vi "OpenLoftyDrve.vi"(8 "error in (no error)":errorcluster) -> (0 "error out":errorcluster)   [LabVIEW 2015]
uses:
  <vilib>/Rock Robotics/WPI/CAN/TalonSRX/WPI_CANTalonSRX_APIControlMode.ctl
  <vilib>/Rock Robotics/WPI/CAN/TalonSRX/WPI_CANTalonSRX_APIFeedbackSelect.ctl
  Advanced Drive VIs/PID Type Def.ctl
  RobotDriveGlobal.vi
  LED Lights/LED Lights Global.vi
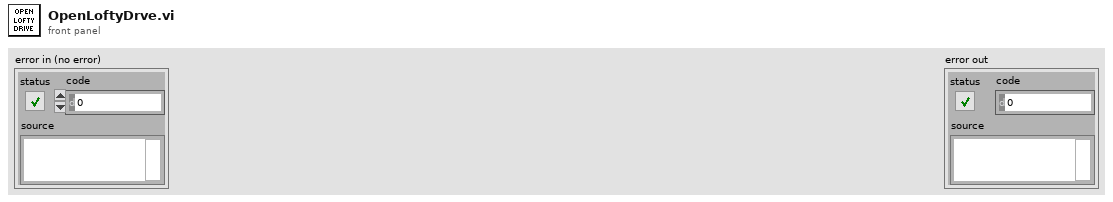
[diagram p1: front panel]
types:
  T1 = typedef "PID Type Def.ctl" = cluster{"P":dbl, "I":dbl, "D":dbl, "F":dbl, "I Zone":dbl, "Ramp Rate":dbl}
  T2 = typedef "WPI_CANTalonSRX_APIFeedbackSelect.ctl" = enum16{"Digital Quadrature Encoder", "Analog Potentiometer", "Analog Encoder", "Count on Quad-A (Rising-Edge)", "Count on Quad-A (Falling-Edge)", "CTR Magnetic Enc (Absolute)", "CTR Magnetic Enc (Relative)", "Pulse Width"}
  T3 = typedef "WPI_CANTalonSRX_APIControlMode.ctl" = enum8{"Percent VBus", "Speed", "Position", "Slave", "Unchanged / Invalid", "Voltage Compensation", "Current", "Motion Profile"}
  T4 = typedef "Drive Global Type Def.ctl" = cluster{"Left Drive Motors":T5, "Right Drive Motors":T5}
  T5 = typedef "Master Slave Drive Motors Type Def.ctl" = cluster{"Motor Front":T6, "Motor Back":T6, "Motor Errors":errorcluster, "Motor Top":T6, "Initialized":bool}
  T6 = typedef "Motor Global Type Def.ctl" = cluster{"Motor Error":errorcluster}
  T7 = typedef "WPI_MotorControlDeviceRef.ctl" = cluster{"DeviceStatus":errorcluster, "Type":T8, "PWM":cluster{"PWM Channel":T9, "DeadBand":T10}, "CAN":cluster{"Device Number":u8, "Control Mode":T11, "Semaphore":T12, "Max Vout":dbl, "TalonSRX Control Mode":T3}, "Invert":bool}
  T8 = typedef "WPI_MotorControlType.ctl" = enum16{"PWM", "CAN", "CANTalonSRX"}
  T9 = typedef "FPGA_DIOPWMChannel.ctl" = enum8{"PWM 0", "PWM 1", "PWM 2", "PWM 3", "PWM 4", "PWM 5", "PWM 6", "PWM 7", "PWM 8", "PWM 9", "PWM MXP 0", "PWM MXP 1", "PWM MXP 2", "PWM MXP 3", "PWM MXP 4", "PWM MXP 5", "PWM MXP 6", "PWM MXP 7", "PWM MXP 8", "PWM MXP 9", "Invalid"}
  T10 = typedef "WPI_PWMDeadband.ctl" = cluster{"Name":string, "maxPositivePwm":i32, "minPositivePwm":i32, "centerPwm":i32, "maxNegativePwm":i32, "minNegativePwm":i32, "angularRange":u16}
  T11 = typedef "WPI_CANJaguar_ControlMode.ctl" = enum8{"Percent VBus", "Current", "Speed", "Position", "Voltage"}
  T12 = typedef "Semaphore RefNum" = refnum<k1>
  T13 = typedef "RobotDrive Type Def.ctl" = cluster{"RobotDriveDevRef":cluster{"DevStatus":errorcluster, "Motors[]":T7[], "Square Inputs":bool, "Max Output":dbl}, "Control Mode":T3, "Motor Settings":T14, "Default Control Mode":T3, "Speed Mag":dbl}
  T14 = typedef "Drive Motor Settings.ctl" = cluster{"Wheel Radius":dbl, "Encoder Ticks Per Rev":dbl, "Gear Ratio":dbl, "ClimbRev":dbl}
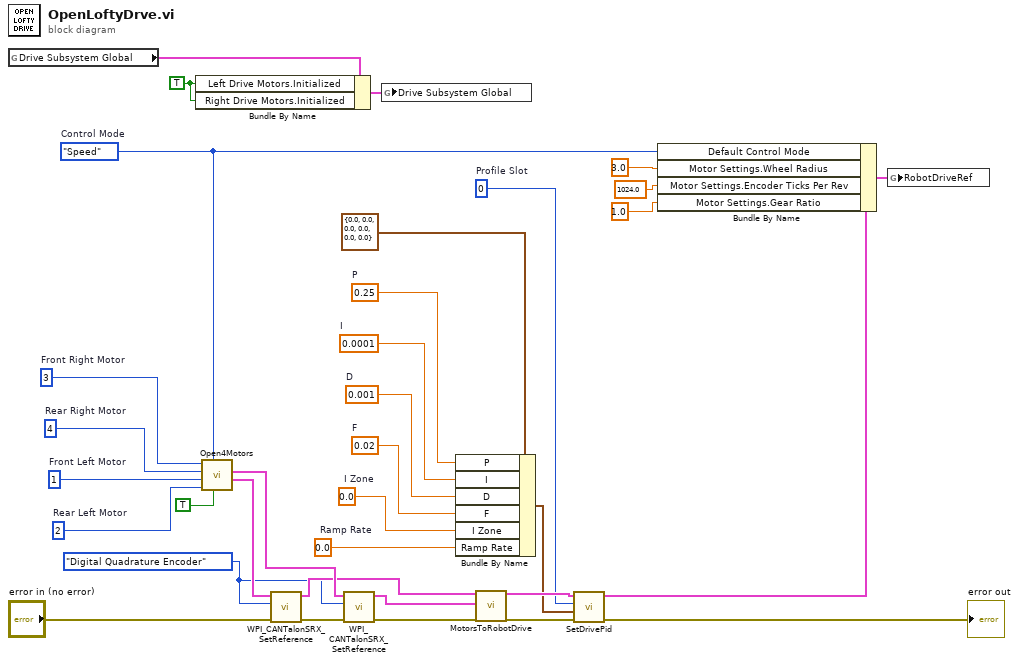
[diagram p0: block diagram]
diagram:
  w34 = TRUE
  w26 = u8 0  # Profile Slot
  w25 = 0.0  # Ramp Rate
  w24 = 0.0  # I Zone
  w23 = 0.02  # F
  w22 = 0.001  # D
  w21 = 0.0001  # I
  w20 = 0.25  # P
  w7 = WPI_CANTalonSRX_APIFeedbackSelect."Digital Quadrature Encoder" ("Feedback Reference")
  w4 = WPI_CANTalonSRX_APIControlMode."Speed"  # Control Mode
  w12 = u8 3  # Front Right Motor
  w14 = u8 1  # Front Left Motor
  w13 = u8 4  # Rear Right Motor
  w15 = u8 2  # Rear Left Motor
  n1 = global read "LED Lights Global.vi" "Drive Subsystem Global"() -> (w3:T4)
  n2 = Bundle By Name(cluster=w3, "Left Drive Motors.Initialized"=w34, "Right Drive Motors.Initialized"=w34) -> (w2:T4)
  n3 = call "Open4Motors.vi"("Invert"=TRUE, "Control Mode"=w4, "Rear Left Device Number"=w15, "Front Left Device Number"=w14, "Rear Right Device Number"=w13, "Front Right Device Number"=w12) -> ("Left Motor"=w18:T7, "Right Motor"=w17:T7)  [unwired: 4 in]
  n4 = call <vilib>:"WPI_CANTalonSRX_SetReference.vi"("error in (no error)"="error in (no error)", "Feedback Reference"=w7, "CAN Talon SRX Ref"=w18) -> ("error out"=w30:errorcluster, "CAN Talon SRX Ref"=w10:T7)  [unwired: 7 in]
  n5 = call <vilib>:"WPI_CANTalonSRX_SetReference.vi"("error in (no error)"=w30, "Feedback Reference"=w7, "CAN Talon SRX Ref"=w17) -> ("error out"=w31:errorcluster, "CAN Talon SRX Ref"=w11:T7)  [unwired: 7 in]
  n6 = global write "LED Lights Global.vi" "Drive Subsystem Global"(w2) -> ()
  n7 = Bundle By Name(cluster=T1 {"P"=0.0, "I"=0.0, "D"=0.0, "F"=0.0, "I Zone"=0.0, "Ramp Rate"=0.0} ("PID"), "P"=w20, "I"=w21, "D"=w22, "F"=w23, "I Zone"=w24, "Ramp Rate"=w25) -> (w27:T1)
  n8 = call "MotorsToRobotDrive.vi"("Left"=w10, "Right"=w11, "error in"=w31) -> ("RobotDriveRef"=w28:T13, "error out"=w32:errorcluster)  [unwired: 15 in]
  n9 = call "SetDrivePid.vi"("error in (no error)"=w32, "PID"=w27, "Profile Slot"=w26, "RobotDriveRef In"=w28) -> ("error out"=→"error out":errorcluster, "RobotDriveRef Out"=w5:T13)  [unwired: 6 in]
  n10 = Bundle By Name(cluster=w5, "Default Control Mode"=w4, "Motor Settings.Wheel Radius"=3.0 ("Wheel Radius"), "Motor Settings.Encoder Ticks Per Rev"=1024.0 ("Encoder Ticks Per Rev"), "Motor Settings.Gear Ratio"=1.0) -> (w1:T13)
  n11 = global write "RobotDriveGlobal.vi" "RobotDriveRef"(w1) -> ()
